vi "Read Spec Page Path.vi"(8 "error in (no error)":errorcluster, 11 "PluginMetaDataObj in":refnum<class "PluginMetaDataObj.lvclass">) -> (0 "error out":errorcluster, 2 "Path to Spec Page VI":path, 3 "PluginMetaDataObj out":refnum<class "PluginMetaDataObj.lvclass">)   [LabVIEW 2020, in "PluginMetaDataObj.lvclass"]
uses:
  PluginMetaDataObj.lvclass
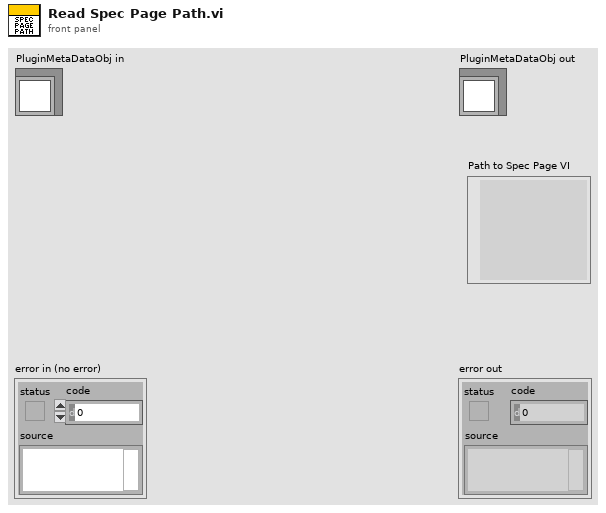
[diagram p1: front panel]
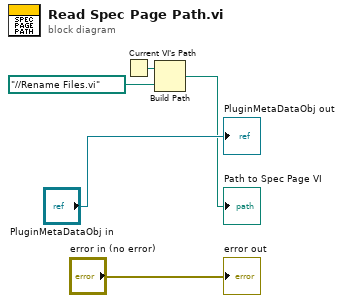
[diagram p0: block diagram]
diagram:
  n1 = Current VI's Path() -> (path=w3:path)
  n2 = Build Path(base path=w3, name or relative path=path "../../Rename Files.vi" ("path")) -> (appended path=→"Path to Spec Page VI":path)
  "error out" <- "error in (no error)"
  "PluginMetaDataObj out" <- "PluginMetaDataObj in"
